vi "Get Data Version.vi"(8 "error in (no error)":errorcluster, 11 "UDPlog Thread Configuration in":refnum<class "UDPlog Thread Configuration.lvclass">) -> (0 "error out":errorcluster, 2 "data version":T1, 3 "UDPlog Thread Configuration out":refnum<class "UDPlog Thread Configuration.lvclass">)   [LabVIEW 2023, in "UDPlog.lvlib" / "UDPlog Thread Configuration.lvclass"]
uses:
  UDPlog Thread Configuration.lvclass
  Users/Public/Documents/National Instruments/NI VeriStand 2023/Custom Devices/Data Sharing Framework/Linux_x64/DSF Core.lvlibp/Typedefs/DSF Version Info.ctl
  Users/Public/Documents/National Instruments/NI VeriStand 2023/Custom Devices/Data Sharing Framework/Linux_x64/DSF Core.lvlibp/Classes/Configuration/Configuration.lvclass
  Users/Public/Documents/National Instruments/NI VeriStand 2023/Custom Devices/Data Sharing Framework/Linux_x64/DSF Core.lvlibp
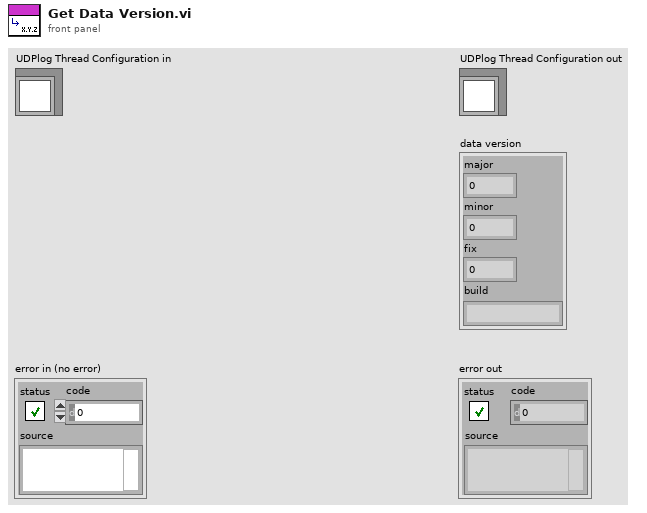
[diagram p1: front panel]
types:
  T1 = typedef "DSF Core.lvlibp/DSF Version Info.ctl" = cluster{"major":u32, "minor":u32, "fix":u32, "build":string}
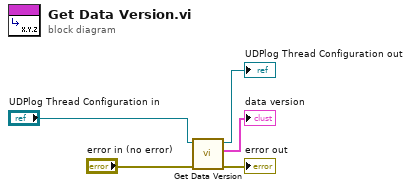
[diagram p0: block diagram]
diagram:
  n1 = call-parent "Get Data Version.vi"("error in (no error)"="error in (no error)", "Configuration in"="UDPlog Thread Configuration in") -> ("error out"=→"error out":errorcluster, "data version"=→"data version":T1, "Configuration out"=→"UDPlog Thread Configuration out":refnum<class "UDPlog Thread Configuration.lvclass">)  [unwired: 7 in]
